vi "movement forward by santimeters.vi"(8 "error in (no error)":errorcluster, 11 "distance (cm)":dbl format="%#_13g") -> (0 "error out":errorcluster)   [LabVIEW 2017]
uses:
  <vilib>/myRIO/Common/Instrument Driver Framework/myRIO v1.0/Encoder/typedefs/Encoder Signal Mode.ctl
  <vilib>/myRIO/Instrument Drivers/Onboard IO/Encoder/typedefs/Encoder Reference.ctl
  <vilib>/myRIO/Common/Instrument Driver Framework/Utilities/typedefs/myRIO Generic Hardware Reference.ctl
  <vilib>/myRIO/Common/Instrument Driver Framework/Utilities/typedefs/Hardware Version Enum.ctl
  <vilib>/myRIO/Common/Instrument Driver Framework/Utilities/typedefs/myRIO v1.0 Reference.ctl
  <vilib>/myRIO/Common/Instrument Driver Framework/Utilities/typedefs/Generic FPGA Reference.ctl
  <vilib>/myRIO/Common/Instrument Driver Framework/myRIO v1.0/Encoder/typedefs/Encoder Channels Enum.ctl
  <vilib>/myRIO/Common/Instrument Driver Framework/myRIO v1.0/Encoder/typedefs/Encoder Configuration v1.0.ctl
  <vilib>/userdefined/High Color/nirio_resource_hc.ctl
  <vilib>/myRIO/Instrument Drivers/Onboard IO/I2C/typedefs/I2C Reference.ctl
  <vilib>/myRIO/Common/Instrument Driver Framework/myRIO v1.0/I2C/typedefs/I2C Channels Enum.ctl
  <vilib>/myRIO/Instrument Drivers/Onboard IO/I2C/typedefs/I2C Configuration.ctl
  <vilib>/myRIO/Instrument Drivers/Onboard IO/I2C/typedefs/I2C Transfer Rate.ctl
  <vilib>/myRIO/Common/Instrument Driver Framework/Utilities/vis/Is FPGA Ref Available.vi
  <vilib>/myRIO/Common/Instrument Driver Framework/myRIO v1.0/Encoder/vis/myRIO v1.1 Open Encoder.vi
  <vilib>/myRIO/Instrument Drivers/Onboard IO/Encoder/vis/Read.vi
  <vilib>/myRIO/Common/Instrument Driver Framework/myRIO v1.0/I2C/vis/myRIO v1.1 Open I2C.vi
  <vilib>/myRIO/Common/Instrument Driver Framework/Utilities/vis/Validate Channels.vi
  <vilib>/myRIO/Common/Instrument Driver Framework/myRIO v1.0/Encoder/vis/myRIO v1.0 Reserve Encoder.vi
  <vilib>/myRIO/Common/Instrument Driver Framework/myRIO v1.0/I2C/vis/myRIO v1.0 Reserve I2C.vi
  <vilib>/myRIO/Common/Instrument Driver Framework/myRIO v1.0/I2C/vis/myRIO v1.0 Close I2C.vi
  <vilib>/myRIO/Common/Instrument Driver Framework/myRIO v1.0/Encoder/vis/myRIO v1.0 Build MUX Configuration Encoder.vi
  <vilib>/myRIO/Common/Instrument Driver Framework/myRIO v1.0/Resource Manager/vis/myRIO v1.0 Reserve Channel List.vi
  <vilib>/myRIO/Common/Instrument Driver Framework/myRIO v1.0/I2C/vis/myRIO v1.0 Build MUX Configuration I2C.vi
  <vilib>/myRIO/Common/Instrument Driver Framework/myRIO v1.0/I2C/vis/myRIO v1.0 Unreserve I2C.vi
  <vilib>/myRIO/Common/Instrument Driver Framework/myRIO v1.0/Resource Manager/vis/myRIO v1.0 Create Configuration List.vi
  <vilib>/myRIO/Common/Instrument Driver Framework/myRIO v1.0/Resource Manager/vis/myRIO v1.0 Reserve Channel.vi
  <vilib>/myRIO/Common/Instrument Driver Framework/myRIO v1.0/Resource Manager/vis/myRIO v1.0 Unreserve Channel.vi
  <vilib>/myRIO/Common/Instrument Driver Framework/myRIO v1.0/Resource Manager/vis/myRIO v1.0 Unreserve Channel List.vi
  <vilib>/myRIO/Common/Instrument Driver Framework/myRIO v1.0/Resource Manager/vis/myRIO v1.0 Build Mutex Name.vi
  <vilib>/Utility/VariantDataType/GetNumericInfo.vi
  <vilib>/Utility/error.llb/Error Cluster From Error Code.vi
  <vilib>/myRIO/Common/Instrument Driver Framework/myRIO v1.0/myRIO v1.1 Open.vi
  <vilib>/myRIO/Common/Instrument Driver Framework/Utilities/vis/IO Manager.vi
  <vilib>/myRIO/Common/Instrument Driver Framework/Utilities/vis/Configuration Manager.vi
  <vilib>/myRIO/Common/Instrument Driver Framework/myRIO v1.0/Resource Manager/vis/myRIO v1.0 Configure IO.vi
  <vilib>/myRIO/Common/Instrument Driver Framework/myRIO v1.0/myRIO v1.0 Close.vi
  <vilib>/myRIO/Common/Instrument Driver Framework/myRIO v1.0/Encoder/vis/myRIO v1.0 Configure Encoder.vi
  <vilib>/myRIO/Common/Instrument Driver Framework/myRIO v1.0/Encoder/vis/myRIO v1.0 Read Encoder.vi
  <vilib>/myRIO/Common/Instrument Driver Framework/myRIO v1.0/DIO/vis/myRIO v1.0 Write DIO.vi
  <vilib>/myRIO/Common/Instrument Driver Framework/myRIO v1.0/I2C/vis/myRIO v1.0 Shutdown I2C.vi
  <vilib>/myRIO/Instrument Drivers/Onboard IO/I2C/vis/myRIO I2C Open.xnode
  <vilib>/myRIO/Express VI/Onboard IO/Encoder/Encoder Express VI.xnode
  <vilib>/myRIO/Instrument Drivers/Onboard IO/Encoder/vis/myRIO Encoder Open.xnode
  <vilib>/myRIO/Instrument Drivers/Onboard IO/I2C/I2C.lvlib
  <vilib>/myRIO/Instrument Drivers/Onboard IO/Encoder/Encoder.lvlib
  <vilib>/myRIO/Instrument Drivers/Onboard IO/DIO/DIO.lvlib
panel:
  out "main angle":ext
  out "axis Z(after)":ext
  out "zero angle":ext
  out "left":dbl
  out "right":dbl
  out "axis Z(paste)":ext
  in  "Stop Button":bool
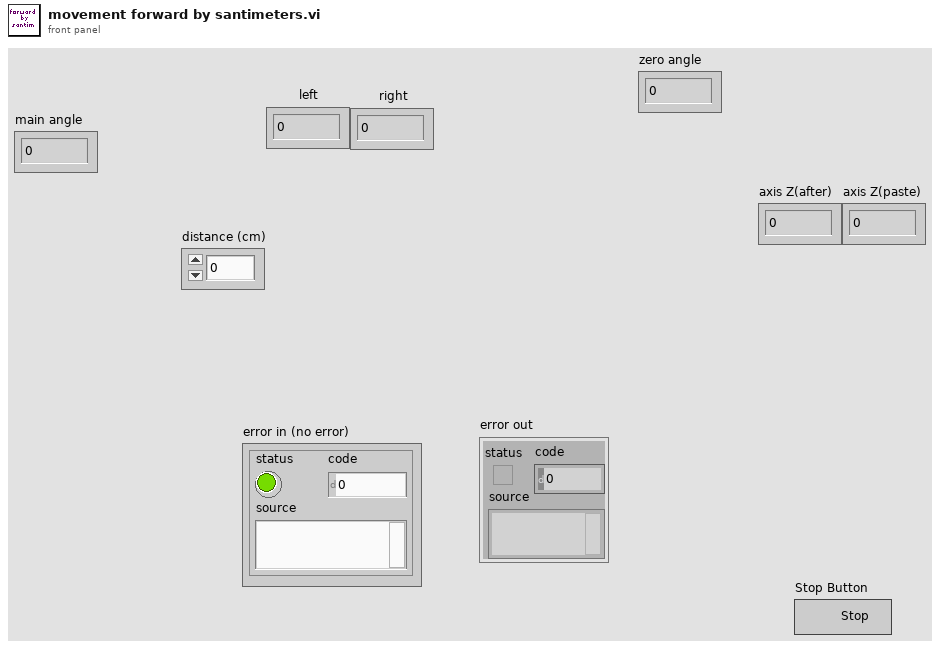
[diagram p1: front panel]
types:
  T1 = typedef "DIO.lvlib/DIO Reference.ctl" = cluster{"myRIO Reference":T2, "DIO Channels List":T6}
  T2 = typedef "myRIO Generic Hardware Reference.ctl" = cluster{"myRIO Model":T3, "myRIO Hardware Reference":T4}
  T3 = typedef "Hardware Version Enum.ctl" = enum16{"Unknown", "myRIO-1900", "myRIO-1950", "roboRIO", "NI ELVIS RIO CM"}
  T4 = typedef "myRIO v1.0 Reference.ctl" = cluster{"Generic FPGA Reference":T5, "Allow multiple opens":bool}
  T5 = typedef "Generic FPGA Reference.ctl" = refnum<k20>
  T6 = typedef "DIO Channels List.ctl" = T7[]
  T7 = typedef "DIO Channels Enum.ctl" = enum16{"Not Connected", "C/DIO0", "C/DIO1", "C/DIO2", "C/DIO3", "C/DIO4", "C/DIO5", "C/DIO6", "C/DIO7", "A/DIO0", "A/DIO1", "A/DIO2", "A/DIO3", "A/DIO4", "A/DIO5", "A/DIO6", "A/DIO7", "A/DIO8", "A/DIO9", "A/DIO10", "A/DIO11", "A/DIO12", "A/DIO13", "A/DIO14", "A/DIO15", "B/DIO0", "B/DIO1", "B/DIO2", "B/DIO3", "B/DIO4", "B/DIO5", "B/DIO6", "B/DIO7", "B/DIO8", "B/DIO9", "B/DIO10", "B/DIO11", "B/DIO12", "B/DIO13", "B/DIO14", "B/DIO15", "LED0", "LED1", "LED2", "LED3", "Button0", "DIO/DIO0", "DIO/DIO1", "DIO/DIO2", "DIO/DIO3", "DIO/DIO4", "DIO/DIO5", "DIO/DIO6", "DIO/DIO7", "DIO/DIO8", "DIO/DIO9", "SPI/CS0", "SPI/CS1", "SPI/CS2", "SPI/CS3", "LED RADIO (Green)", "LED RADIO (Red)", "LED COMM (Green)", "LED COMM (Red)", "LED MODE (Green)", "LED MODE (Red)"}
  T8 = typedef "I2C.lvlib/I2C Reference.ctl" = cluster{"myRIO Reference":T2, "I2C Channels Enum":T9, "I2C Configuration":T10}
  T9 = typedef "I2C Channels Enum.ctl" = enum16{"Not Connected", "A/I2C", "B/I2C", "I2C/I2C"}
  T10 = typedef "I2C.lvlib/I2C Configuration.ctl" = cluster{"I2C Transfer Rate":T11}
  T11 = typedef "I2C.lvlib/I2C Transfer Rate.ctl" = enum16{"Standard mode (100 kbps)", "Fast mode (400 kbps)"}
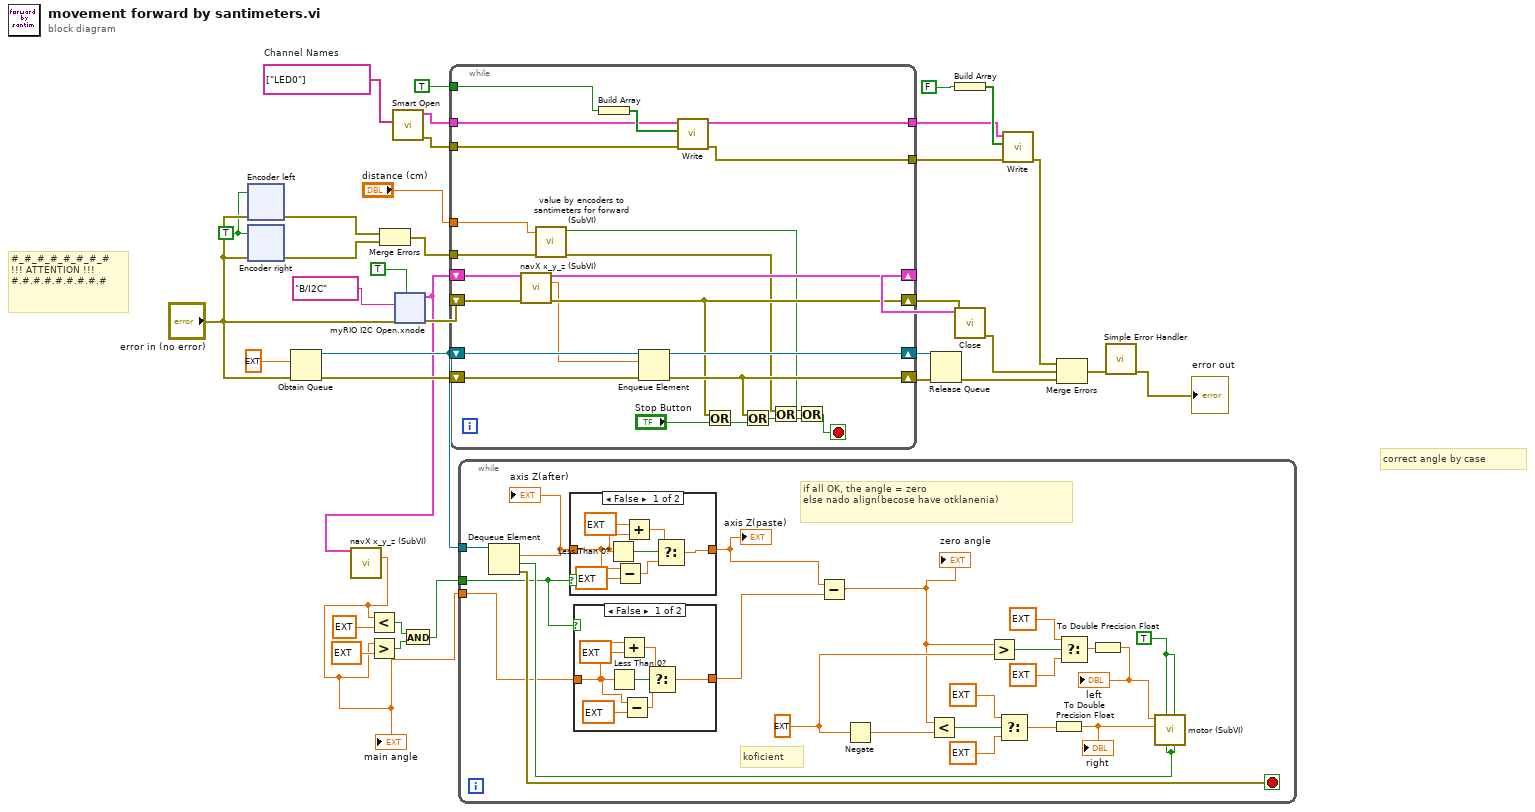
[diagram p0: block diagram]
diagram:
  w9 = tag[] ["LED0"]  # Channel Names
  w10 = TRUE ("Reset Counter")
  # "correct angle by case"
  # "#_#_#_#_#_#_#_#\n!!! ATTENTION !!!\n#.#.#.#.#.#.#.#.#"
  n1 = xnode ("Encoder left")("error in (no error)"="error in (no error)", "Reset Counter"=w10) -> ("error out"=w14:errorcluster)  [unwired: 3 out]
  n2 = xnode ("Encoder right")("error in (no error)"="error in (no error)", "Reset Counter"=w10) -> ("error out"=w13:errorcluster)  [unwired: 3 out]
  n3 = Obtain Queue(element data type=ext 0.0 ("value Z"), error in (no error)="error in (no error)") -> (queue out=w24:refnum<queue>, error out=w36:errorcluster)  [unwired: 3 in, 1 out]
  n4 = Merge Errors(w14, w13) -> (w12:errorcluster)
  n5 = call <vilib>:"Smart Open.vi"("Channel Names"=w9) -> ("error out"=w4:errorcluster, "DIO Ref Out"=w5:T1)  [unwired: 9 in]
  n6 = xnode "myRIO I2C Open.xnode"("error in (no error)"="error in (no error)", "Allow multiple opens?"=TRUE, "Channel Name"=tag "B/I2C") -> ("error out"=w29:errorcluster, "I2C Ref Out"=w22:T8)
  n7 = call "navX x_y_z (SubVI).vi"("I2C Ref Out in"=w22) -> ("value Z"=w19:ext)  [unwired: 10 in, 4 out]
  "main angle" <- w19
  n8 = Less?(x=w19, y=ext 90.0) -> (x < y?=w17:bool)
  n9 = Greater?(x=w19, y=ext -90.0) -> (0:w20:bool)
  n10 = And(x=w17, y=w20) -> (x .and. y?=w16:bool)
  n11 = while {
    shift-right: [w54] -> w34
    shift-left: w36 -> [w59]
    shift-right: [w58] -> w35
    shift-left: w24 -> [w60]
    shift-right: [w55] -> w30
    shift-left: w22 -> [w56]
    shift-right: [w51] -> w28
    shift-left: w29 -> [w52]
    tunnel: w12 -> [w46]
    tunnel: "distance (cm)" -> [w44]
    tunnel: TRUE -> [w41]
    tunnel: w5 -> [w40]
    tunnel: w4 -> [w39]
    tunnel: [w38] -> w2
    tunnel: [w37] -> w3
    stop <- w48 stop-if-true
    n12 = call "navX x_y_z (SubVI).vi"("I2C Ref Out in"=w56, "error in (no error)"=w52) -> ("I2C Ref Out out"=w55:T8, "value Z"=w50:ext, "error out"=w51:errorcluster)  [unwired: 9 in, 2 out]
    n13 = call "value by encoders to santimeters for forward (SubVI).vi"("error in (no error)"=w46, "range in"=w44) -> ("error out"=w45:errorcluster, "value >= range"=w43:bool)  [unwired: 7 in, 1 out]
    n14 = Build Array(w41) -> (w42:bool[])
    n15 = Enqueue Element(queue=w60, element=w50, error in (no error)=w59) -> (queue out=w58:refnum<queue>, error out=w54:errorcluster)  [unwired: 1 in, 1 out]
    n16 = call <vilib>:"Write.vi"("error in (no error)"=w39, "Values"=w42, "DIO Ref In"=w40) -> ("error out"=w37:errorcluster, "DIO Ref Out"=w38:T1)  [unwired: 6 in]
    n17 = Or(x=w51, y="Stop Button") -> (x .or. y?=w53:bool)
    n18 = Or(x=w54, y=w53) -> (x .or. y?=w49:bool)
    n19 = Or(x=w45, y=w49) -> (x .or. y?=w47:bool)
    n20 = Or(x=w43, y=w47) -> (x .or. y?=w48:bool)
  }
  n21 = while {
    tunnel: w24 -> [w82]
    tunnel: w19 -> [w64]
    tunnel: w16 -> [w63]
    stop <- w81 stop-if-true
    w70 = TRUE ("M0 (Pin 21)")
    w74 = ext 1.0 ("y")
    # "koficient"
    # "if all OK, the angle = zero\nelse nado align(becose have otklanenia)"
    n22 = Dequeue Element(queue=w82) -> (element=w66:ext, timed out?=w69:bool, error out=w81:errorcluster)  [unwired: 2 in, 1 out]
    "axis Z(after)" <- w66
    n23 = case shown="False" w63 {
      tunnel: [w96 w98] -> w67
      tunnel: w66 -> [w92 w98]
      frame False {
        n24 = Less Than 0?(x=w92) -> (x < 0?=w97:bool)
        n25 = Subtract(x=w92, y=ext 180.0) -> (x-y=w93:ext)
        n26 = Add(x=ext 180.0, y=w92) -> (x+y=w95:ext)
        n27 = Select(t=w95, s=w97, f=w93) -> (s? t:f=w96:ext)
      }
      frame True {
      }
    }
    "axis Z(paste)" <- w67
    n28 = case shown="False" w63 {
      tunnel: [w88 w90] -> w65
      tunnel: w64 -> [w85 w90]
      frame False {
        n29 = Less Than 0?(x=w85) -> (x < 0?=w89:bool)
        n30 = Add(x=w85, y=ext 180.0) -> (x+y=w87:ext)
        n31 = Subtract(x=w85, y=ext 180.0) -> (x-y=w86:ext)
        n32 = Select(t=w87, s=w89, f=w86) -> (s? t:f=w88:ext)
      }
      frame True {
      }
    }
    n33 = Subtract(x=w67, y=w65) -> (x-y=w68:ext)
    "zero angle" <- w68
    n34 = Negate(x=w74) -> (-x=w73:ext)
    n35 = Less?(x=w68, y=w73) -> (x < y?=w77:bool)
    n36 = Greater?(x=w68, y=w74) -> (0:w80:bool)
    n37 = Select(t=ext 0.2 ("y"), s=w77, f=ext 0.30000000000000000001 ("y")) -> (s? t:f=w71:ext)
    n38 = To Double Precision Float(number=w71) -> (double precision float=w62:dbl)
    "right" <- w62
    n39 = Select(t=ext 0.2 ("y"), s=w80, f=ext 0.30000000000000000001 ("y")) -> (s? t:f=w72:ext)
    n40 = To Double Precision Float(number=w72) -> (double precision float=w61:dbl)
    "left" <- w61
    n41 = call "motor (SubVI).vi"("M1 (Pin 26)"=w69, "M1 (Pin 25)"=w70, "M0 (Pin 23)"=w69, "M0 (Pin 21)"=w70, "PWM1"=w62, "PWM0"=w61) -> ()  [unwired: 5 in, 1 out]
  }
  n42 = Release Queue(queue=w35, error in (no error)=w34) -> (error out=w25:errorcluster)  [unwired: 1 in, 2 out]
  n43 = Build Array(FALSE) -> (w8:bool[])
  n44 = call <vilib>:"Close.vi"("error in (no error)"=w28, "I2C Ref In"=w30) -> ("error out"=w26:errorcluster)  [unwired: 9 in]
  n45 = call <vilib>:"Write.vi"("error in (no error)"=w3, "Values"=w8, "DIO Ref In"=w2) -> ("error out"=w1:errorcluster)  [unwired: 6 in, 1 out]
  n46 = Merge Errors(w1, w26, w25) -> (w27:errorcluster)
  n47 = call <vilib>:"Simple Error Handler.vi"("error in (no error)"=w27) -> ("error out"=→"error out":errorcluster)  [unwired: 4 in, 4 out]
